vi "UTIL Predict Class with Variance HMM.vi"(5 "Data Point":dbl[](array[numeric]), 7 "Transition Matrix":dbl[][](array[numeric]), 8 "Cluster Data From File":dbl[][](array[numeric]), 9 "d(t-1) In":dbl[](array[numeric])) -> (2 "Sleep Stage":i32, 3 "d(t-1) Out":dbl[](array[numeric]))   [LabVIEW 2010]
doc: "This VI approximates the current sleep state given a data point. It uses an approximation of conditional probability, the variance normalized distance from a cluster centroid multiplied by the state porbabilities, and assigns the class of maximum probability.\n\nInputs:\n Data Point 1D Array of DBL, Current data point\n in 3D feature space\n Cluster Data From File 2D Array of DBL,MATLAB computed \n centroids and variances of clusters\n\n\nOutputs:\n Sleep Stage SGL, assigned sleep stage prediction"
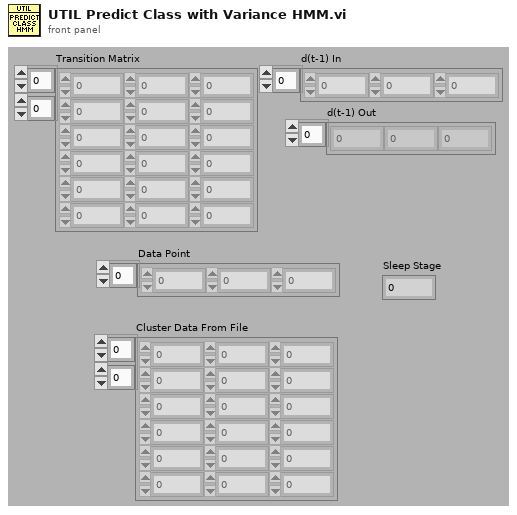
[diagram p1: front panel]
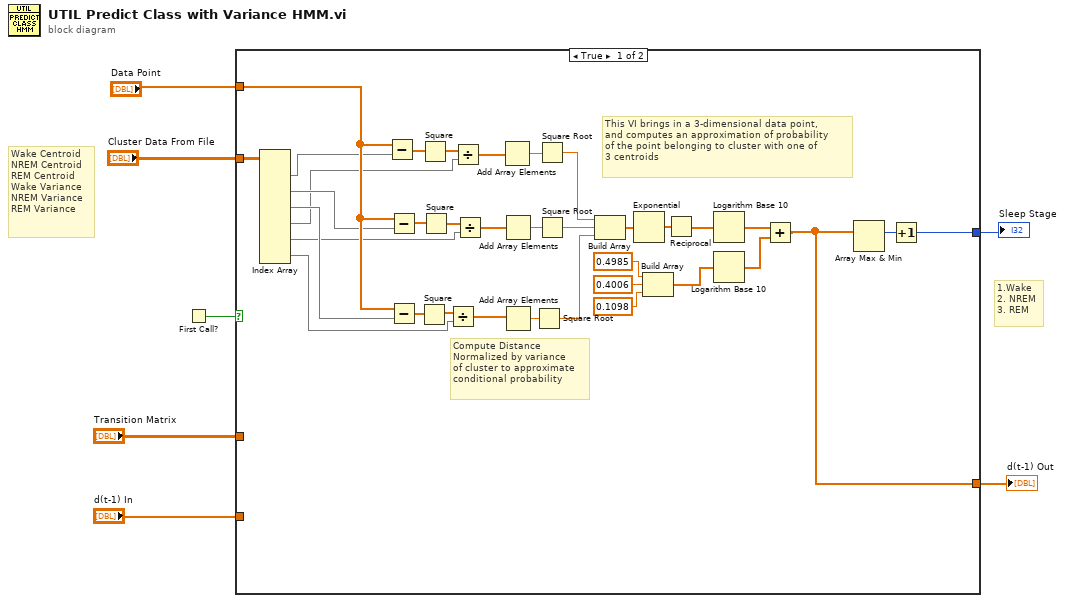
[diagram p0: block diagram]
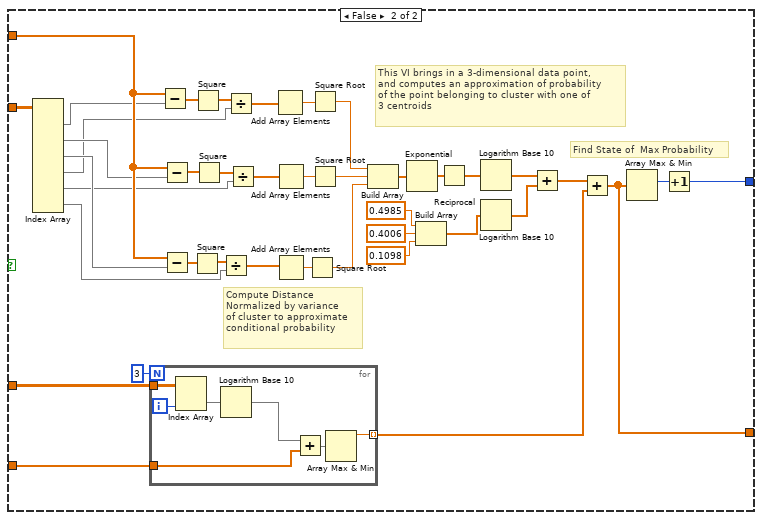
[diagram p2: hidden frame]
diagram:
  # "Wake Centroid\nNREM Centroid\nREM Centroid\nWake Variance\nNREM Variance\nREM Variance"
  # "1.Wake\n2. NREM\n3. REM"
  n1 = First Call?() -> (First Call?: T/F=w1:bool)
  n2 = case shown="True" w1 {
    tunnel: [w42 w82] -> w7
    tunnel: "Data Point" -> [w35 w75]
    tunnel: "Cluster Data From File" -> [w30 w70]
    tunnel: "Transition Matrix" -> [_ w52]
    tunnel: "d(t-1) In" -> [_ w51]
    tunnel: [w11 w50] -> w2
    frame True {
      # "This VI brings in a 3-dimensional data point,\nand computes an approximation of probability\nof the point belonging to cluster with one of \n3 centroids"
      # "Compute Distance\nNormalized by variance \nof cluster to approximate \nconditional probability"
      n3 = Index Array(array=w30) -> (element #1=w31:dbl[], element #2=w29:dbl[], element #3=w28:dbl[], element #4=w17:dbl[], element #5=w21:dbl[], element #6=w25:dbl[])  [unwired: 12 in]
      n4 = Subtract(x=w35, y=w31) -> (x-y=w19:dbl[])
      n5 = Subtract(x=w35, y=w29) -> (x-y=w23:dbl[])
      n6 = Subtract(x=w35, y=w28) -> (x-y=w27:dbl[])
      n7 = Square(x=w27) -> (x^2=w26:dbl[])
      n8 = Square(x=w19) -> (x^2=w18:dbl[])
      n9 = Square(x=w23) -> (x^2=w22:dbl[])
      n10 = Divide(x=w26, y=w25) -> (x/y=w24:dbl[])
      n11 = Divide(x=w18, y=w17) -> (x/y=w16:dbl[])
      n12 = Divide(x=w22, y=w21) -> (x/y=w20:dbl[])
      n13 = Add Array Elements(numeric array=w16) -> (sum=w36:dbl)
      n14 = Add Array Elements(numeric array=w20) -> (sum=w37:dbl)
      n15 = Add Array Elements(numeric array=w24) -> (sum=w38:dbl)
      n16 = Square Root(x=w38) -> (sqrt(x)=w41:dbl)
      n17 = Square Root(x=w36) -> (sqrt(x)=w40:dbl)
      n18 = Square Root(x=w37) -> (sqrt(x)=w39:dbl)
      n19 = Build Array(w40, w39, w41) -> (w34:dbl[])
      n20 = Exponential(1:w34) -> (0:w33:dbl[])
      n21 = Build Array(0.4985, 0.4006, 0.1098) -> (w10:dbl[])
      n22 = Reciprocal(x=w33) -> (1/x=w9:dbl[])
      n23 = Logarithm Base 10(1:w9) -> (0:w8:dbl[])
      n24 = Logarithm Base 10(1:w10) -> (0:w12:dbl[])
      n25 = Add(x=w8, y=w12) -> (x+y=w11:dbl[])
      n26 = Array Max & Min(array=w11) -> (max index (indices)=w32:i32)  [unwired: 3 out]
      n27 = Increment(x=w32) -> (x+1=w42:i32)
    }
    frame False {
      # "Find State of  Max Probability"
      # "This VI brings in a 3-dimensional data point,\nand computes an approximation of probability\nof the point belonging to cluster with one of \n3 centroids"
      # "Compute Distance\nNormalized by variance \nof cluster to approximate \nconditional probability"
      n28 = Index Array(array=w70) -> (element #1=w71:dbl[], element #2=w69:dbl[], element #3=w68:dbl[], element #4=w57:dbl[], element #5=w61:dbl[], element #6=w65:dbl[])  [unwired: 12 in]
      n29 = for {
        N: 3 ("Numeric") -> [_]
        tunnel: w52 -> [w88]
        tunnel: w51 -> [w89]
        tunnel: [w85] -> w43 mode=indexing
        i -> [w84]
        n30 = Index Array(array=w88, index (col)=w84) -> (element=w87:dbl[])  [unwired: 1 in]
        n31 = Logarithm Base 10(1:w87) -> (0:w83:dbl[])
        n32 = Add(x=w83, y=w89) -> (x+y=w86:dbl[])
        n33 = Array Max & Min(array=w86) -> (max value=w85:dbl)  [unwired: 3 out]
      }
      n34 = Subtract(x=w75, y=w71) -> (x-y=w59:dbl[])
      n35 = Subtract(x=w75, y=w69) -> (x-y=w63:dbl[])
      n36 = Subtract(x=w75, y=w68) -> (x-y=w67:dbl[])
      n37 = Square(x=w67) -> (x^2=w66:dbl[])
      n38 = Square(x=w59) -> (x^2=w58:dbl[])
      n39 = Square(x=w63) -> (x^2=w62:dbl[])
      n40 = Divide(x=w66, y=w65) -> (x/y=w64:dbl[])
      n41 = Divide(x=w58, y=w57) -> (x/y=w56:dbl[])
      n42 = Divide(x=w62, y=w61) -> (x/y=w60:dbl[])
      n43 = Add Array Elements(numeric array=w56) -> (sum=w76:dbl)
      n44 = Add Array Elements(numeric array=w60) -> (sum=w77:dbl)
      n45 = Add Array Elements(numeric array=w64) -> (sum=w78:dbl)
      n46 = Square Root(x=w78) -> (sqrt(x)=w81:dbl)
      n47 = Square Root(x=w76) -> (sqrt(x)=w80:dbl)
      n48 = Square Root(x=w77) -> (sqrt(x)=w79:dbl)
      n49 = Build Array(w80, w79, w81) -> (w74:dbl[])
      n50 = Exponential(1:w74) -> (0:w73:dbl[])
      n51 = Build Array(0.4985, 0.4006, 0.1098) -> (w46:dbl[])
      n52 = Reciprocal(x=w73) -> (1/x=w45:dbl[])
      n53 = Logarithm Base 10(1:w45) -> (0:w48:dbl[])
      n54 = Logarithm Base 10(1:w46) -> (0:w47:dbl[])
      n55 = Add(x=w48, y=w47) -> (x+y=w44:dbl[])
      n56 = Add(x=w44, y=w43) -> (x+y=w50:dbl[])
      n57 = Array Max & Min(array=w50) -> (max index (indices)=w72:i32)  [unwired: 3 out]
      n58 = Increment(x=w72) -> (x+1=w82:i32)
    }
  }
  "Sleep Stage" <- w7
  "d(t-1) Out" <- w2
